vi "URAPI_End_Subroutine.vi"(3 "URAPI Script in":T1) -> (1 "URAPI Script out":T1)   [LabVIEW 2012]
uses:
  <userlib>/BotSpeak/VIs/Direct/URAPI_Control.ctl
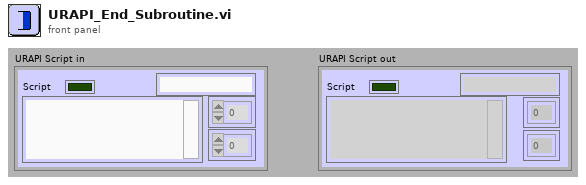
[diagram p1: front panel]
types:
  T1 = typedef "URAPI_Control.ctl" = cluster{"Script":string, "Whiles":u8[], "Ifs":u8[], "Supress Err":bool, "Errors":string}
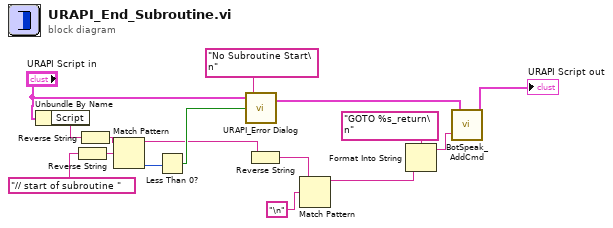
[diagram p0: block diagram]
diagram:
  n1 = Unbundle By Name("URAPI Script in") -> ("Script"=w15:string)
  n2 = Reverse String(1:"// start of subroutine " ("String")) -> (0:w3:string)
  n3 = Reverse String(1:w15) -> (0:w4:string)
  n4 = Match Pattern(string=w4, regular expression=w3) -> (before substring=w1:string, offset past match=w9:i32)  [unwired: 1 in, 2 out]
  n5 = Less Than 0?(x=w9) -> (x < 0?=w8:bool)
  n6 = call <userlib>:"URAPI_Error Dialog.vi"("Error String"="No Subroutine Start\n" ("String"), "Error?"=w8, "URAPI Script in"="URAPI Script in") -> ("URAPI Script out"=w7:T1)  [unwired: 1 in]
  n7 = Reverse String(1:w1) -> (0:w2:string)
  n8 = Match Pattern(string=w2, regular expression="\n" ("String")) -> (before substring=w12:string)  [unwired: 1 in, 3 out]
  n9 = Format Into String(format string="GOTO %s_return\n" ("String"), w12) -> (resulting string=w11:string)  [unwired: 2 in, 1 out]
  n10 = call <userlib>:"BotSpeak_AddCmd.vi"("String"=w11, "URAPI Script"=w7) -> ("URAPI Script out"=→"URAPI Script out":T1)  [unwired: 1 in]
